vi "Configure Marker Destination.vi"(6 "Alternate Amplitude (0: None)":u16(ring) items=["None", "Marker1", "Marker2", "Marker3", "Marker4"], 7 "Pulse (0: None)":u16(ring) items=["None", "Marker1", "Marker2", "Marker3", "Marker4"], 8 "error in (no error)":errorcluster, 9 "ALC Hold (0: None)":u16(ring) items=["None", "Marker1", "Marker2", "Marker3", "Marker4"], 10 "Modulation Format (1: Dual Modulation)":u16(ring)=1 items=["Dual Modulation"=1, "Dual ARB"=2, "Multitone"=3, "Two-tone"=6, "AWGN ARB"=8], 11 "VISA resource name":refnum<visa-resource-name>) -> (0 "error out":errorcluster, 3 "VISA resource name out":refnum<visa-resource-name>)   [LabVIEW 2009, in "Agilent PSG MXG Series.lvlib"]
doc: "Configures the marker pulse/RF function, ALC hold function and alternate amplitude for the specific modulation format.\n\n<B>Notes:</B>\n(1) This VI is valid only in E8267C, E8257D, E8267D, N5182A.\n\n(2) For E8267C, this VI is valid only when the instrument installs <B>Option 002</B> (Internal baseband generator) or <B>Option 602</B> (Digital bus baseband generator).\n\n(3) For E8267D, this VI is valid only when the instrument installs <B>Option 601</B> or <B>Option 602</B> (Internal baseband generator).\n\n(4) For N5182A, this VI is valid only when the instrument installs <B>Option 651</B> or <B>Option 652</B> or <B>Option 654</B> (Internal baseband generator), and <B>Option 432</B> (Phase noise impairment)."
uses:
  Agilent PSG MXG Series.lvlib
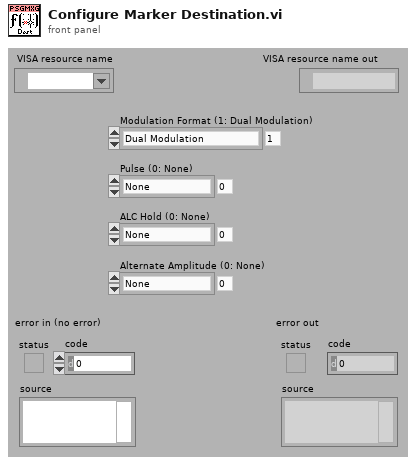
[diagram p1: front panel]
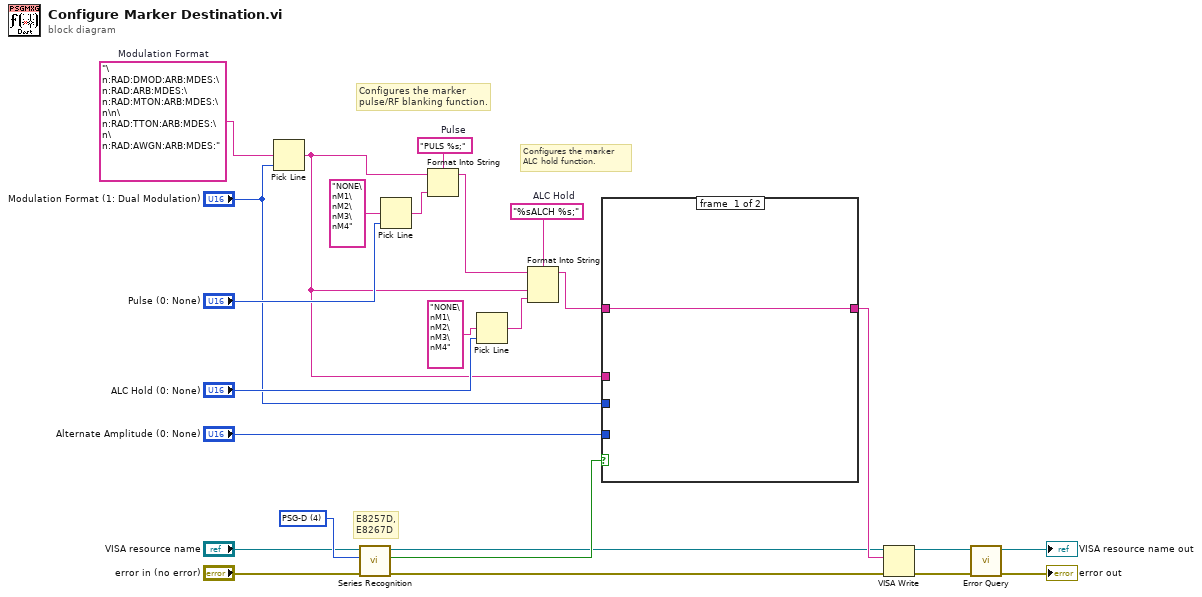
[diagram p0: block diagram]
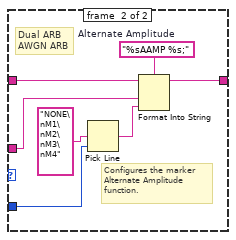
[diagram p3: hidden frame]
diagram:
  w14 = u16 4 items=["MXG", "PSG", "PSG-A", "PSG-C", "PSG-D"] ("Series Type (0: MXG)")
  w19 = "%sALCH %s;"  # ALC Hold
  w24 = "PULS %s;"  # Pulse
  w25 = "\n:RAD:DMOD:ARB:MDES:\n:RAD:ARB:MDES:\n:RAD:MTON:ARB:MDES:\n\n\n:RAD:TTON:ARB:MDES:\n\n:RAD:AWGN:ARB:MDES:"  # Modulation Format
  # "E8257D,\nE8267D"
  # "Configures the marker\nALC hold function."
  # "Configures the marker\npulse/RF blanking function."
  n1 = Pick Line(multi-line string=w25, line index="Modulation Format (1: Dual Modulation)") -> (output string=w8:string)  [unwired: 1 out]
  n2 = call "Series Recognition.vi"("error in (no error)"="error in (no error)", "Series Type (0: MXG)"=w14, "VISA resource name"="VISA resource name") -> ("error out"=w5:errorcluster, "Is Series Correct"=w13:bool, "VISA resource name out"=w6:refnum<visa-resource-name>)  [unwired: 6 out]
  n3 = Pick Line(multi-line string="NONE\nM1\nM2\nM3\nM4", line index="Pulse (0: None)") -> (output string=w23:string)  [unwired: 1 out]
  n4 = Format Into String(format string=w24, initial string=w8, w23) -> (resulting string=w20:string)  [unwired: 1 in, 1 out]
  n5 = Pick Line(multi-line string="NONE\nM1\nM2\nM3\nM4", line index="ALC Hold (0: None)") -> (output string=w9:string)  [unwired: 1 out]
  n6 = Format Into String(format string=w19, initial string=w20, w8, w9) -> (resulting string=w11:string)  [unwired: 1 in, 1 out]
  n7 = case shown="True" w13 {
    tunnel: "Modulation Format (1: Dual Modulation)" -> [_ w31]
    tunnel: w11 -> [w26 w30]
    tunnel: "Alternate Amplitude (0: None)" -> [_ w29]
    tunnel: w8 -> [_ w28]
    tunnel: [w26 w27] -> w7
    frame #0 {
    }
    frame #1 {
      # "PSG-D"
      n8 = case shown="2, 8" w31 {
        tunnel: w30 -> [w32 w36]
        tunnel: w29 -> [_ w35]
        tunnel: w28 -> [_ w34]
        tunnel: [w32 w33] -> w27
        frame #0 {
        }
        frame #1 {
          w39 = "%sAAMP %s;"  # Alternate Amplitude
          # "Dual ARB\nAWGN ARB"
          # "Configures the marker\nAlternate Amplitude\nfunction."
          n9 = Pick Line(multi-line string="NONE\nM1\nM2\nM3\nM4", line index=w35) -> (output string=w38:string)  [unwired: 1 out]
          n10 = Format Into String(format string=w39, initial string=w36, w34, w38) -> (resulting string=w33:string)  [unwired: 1 in, 1 out]
        }
      }
    }
  }
  n11 = VISA Write(VISA resource name=w6, write buffer=w7, error in (no error)=w5) -> (VISA resource name out=w16:refnum<visa-resource-name>, error out=w15:errorcluster)  [unwired: 1 out]
  n12 = call "Error Query.vi"("error in (no error)"=w15, "VISA resource name"=w16) -> ("error out"=→"error out":errorcluster, "VISA resource name out"=→"VISA resource name out":refnum<visa-resource-name>)  [unwired: 8 out]
